vi "get_led_array.vi"(11 "y":i32) -> (3 "Array":bool[](array[boolean]))   [LabVIEW 2022 SP3]
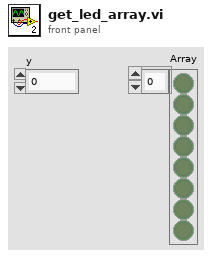
[diagram p1: front panel]
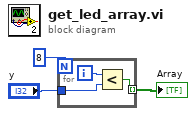
[diagram p0: block diagram]
diagram:
  n1 = for {
    N: 8 -> [_]
    tunnel: "y" -> [w5]
    tunnel: [w4] -> w3 mode=indexing
    i -> [w6]
    n2 = Less?(x=w6, y=w5) -> (x < y?=w4:bool)
  }
  "Array" <- w3
